vi "IHM_SetNumericValue.vi"(4 "error in (no error)":errorcluster caption="entrée d'erreur (pas d'erreur)", 6 "NumericValue":i32, 7 "Ref_IN":T1) -> (0 "Error out":errorcluster, 3 "Ref_OUT":T1)   [LabVIEW 2013]
panel:
  out "ClassName":string
  out "Name":string
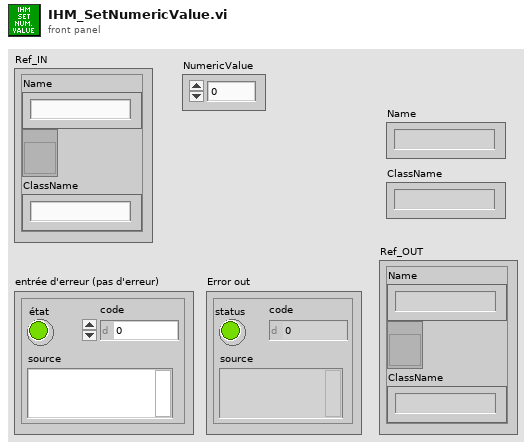
[diagram p1: front panel]
types:
  T1 = cluster{"Name":string, refnum<vi>, "ClassName":string}
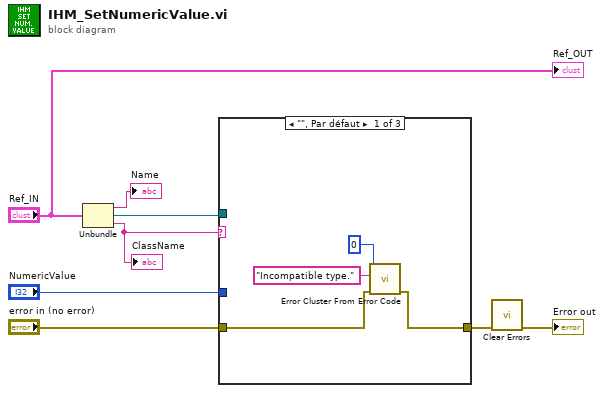
[diagram p0: block diagram]
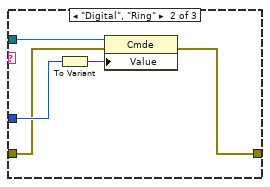
[diagram p2: hidden frame]
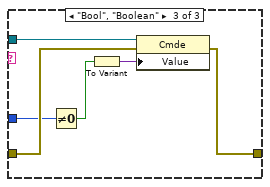
[diagram p3: hidden frame]
diagram:
  n1 = Unbundle("Ref_IN") -> ("Name"=→"Name":string, w7:refnum<vi>, "ClassName"=w8:string)
  "ClassName" <- w8
  n2 = case shown="\"\", Par défaut" w8 {
    tunnel: w7 -> [_ w17 w23]
    tunnel: "error in (no error)" -> [w12 w14 w21]
    tunnel: [w11 w13 w20] -> w2
    tunnel: "NumericValue" -> [_ w15 w19]
    frame "", Default {
      n3 = call <vilib>:"Error Cluster From Error Code.vi"("error in (no error)"=w12, "error message (\"\")"="Incompatible type." ("error message (\"\")"), "error code (0)"=0) -> ("error out"=w11:errorcluster)  [unwired: 6 in]
    }
    frame "Digital", "Ring" {
      n4 = To Variant(anything=w15) -> (Variant=w16:variant)
      n5 = property class="Cmde"(reference=w17, error in=w14, "Value"=w16) -> (error out=w13:errorcluster)  [unwired: 1 out]
    }
    frame "Bool", "Boolean" {
      n6 = Not Equal To 0?(x=w19) -> (x != 0?=w18:bool)
      n7 = To Variant(anything=w18) -> (Variant=w22:variant)
      n8 = property class="Cmde"(reference=w23, error in=w21, "Value"=w22) -> (error out=w20:errorcluster)  [unwired: 1 out]
    }
  }
  n9 = call <vilib>:"Clear Errors.vi"("error in (no error)"=w2) -> ("error out"=→"Error out":errorcluster)  [unwired: 6 in]
  "Ref_OUT" <- "Ref_IN"
